vi "S7-PPI协议.vi"() -> ()   [LabVIEW 2014]
uses:
  <vilib>/Platform/browser.llb/Open URL in Default Browser (string).vi
  <vilib>/Instr/_visa.llb/VISA Configure Serial Port (Instr).vi
panel:
  out "RVW34":u16
  out "RVW32":u16
  out "RVW30":u16
  out "RVW28":u16
  out "RVW26":u16
  out "RVW24":u16
  out "RVW22":u16
  out "RVW20":u16
  out "RVW18":u16
  out "RVW16":u16
  out "RVW14":u16
  out "RVW12":u16
  out "RVW10":u16
  out "RVW8":u16
  out "RVW6":u16
  out "RVW4":u16
  out "RVW2":u16
  out "RVW0":u16
  in  "VW34":u16
  in  "VW32":u16
  in  "VW30":u16
  in  "VW28":u16
  in  "VW26":u16
  in  "VW24":u16
  in  "VW22":u16
  in  "VW20":u16
  in  "VW18":u16
  in  "VW16":u16
  in  "VW14":u16
  in  "VW12":u16
  in  "VW10":u16
  in  "VW8":u16
  in  "VW6":u16
  in  "VW4":u16
  in  "VW2":u16
  in  "VW0":u16
  out "值 3":u32
  out "Q3.0":bool
  out "Q3.1":bool
  out "Q3.2":bool
  out "Q3.3":bool
  out "Q3.4":bool
  out "Q3.5":bool
  out "Q3.6":bool
  out "Q3.7":bool
  out "M2.0":bool
  out "M2.1":bool
  out "M2.2":bool
  out "M2.4":bool
  out "M2.3":bool
  out "M2.5":bool
  out "M2.6":bool
  out "M2.7":bool
  out "M1.0":bool
  out "M1.1":bool
  out "M1.2":bool
  out "M1.3":bool
  out "M1.4":bool
  out "M1.5":bool
  out "M1.6":bool
  out "M1.7":bool
  out "M0.0":bool
  out "M0.1":bool
  out "M0.2":bool
  out "M0.3":bool
  out "M0.4":bool
  out "M0.5":bool
  out "M0.6":bool
  out "M0.7":bool
  in  "Q3.0":bool
  in  "Q3.1":bool
  in  "Q3.2":bool
  in  "Q3.3":bool
  in  "Q3.4":bool
  in  "Q3.5":bool
  in  "Q3.6":bool
  in  "Q3.7":bool
  in  "M2.0":bool
  in  "M2.1":bool
  in  "M2.2":bool
  in  "M2.3":bool
  in  "M2.4":bool
  in  "M2.5":bool
  in  "M2.6":bool
  in  "M2.7":bool
  in  "M1.0":bool
  in  "M1.1":bool
  in  "M1.2":bool
  in  "M1.3":bool
  in  "M1.4":bool
  in  "M1.5":bool
  in  "M1.6":bool
  in  "M1.7":bool
  in  "M0.0":bool
  in  "M0.1":bool
  in  "M0.2":bool
  in  "M0.3":bool
  in  "M0.4":bool
  in  "M0.5":bool
  in  "M0.6":bool
  in  "M0.7":bool
  out "值 2":u32
  in  "Q3.0":bool
  in  "Q3.1":bool
  in  "Q3.2":bool
  in  "Q3.3":bool
  in  "Q3.4":bool
  in  "Q3.5":bool
  in  "Q3.6":bool
  in  "Q3.7":bool
  in  "Q2.0":bool
  in  "Q2.1":bool
  in  "Q2.2":bool
  in  "Q2.3":bool
  in  "Q2.4":bool
  in  "Q2.5":bool
  in  "Q2.6":bool
  in  "Q2.7":bool
  in  "Q1.7":bool
  in  "Q1.6":bool
  in  "Q1.5":bool
  in  "Q1.4":bool
  in  "Q1.3":bool
  in  "Q1.2":bool
  in  "Q1.1":bool
  in  "Q1.0":bool
  in  "Q0.7":bool
  in  "Q0.6":bool
  in  "Q0.5":bool
  in  "Q0.4":bool
  in  "Q0.3":bool
  in  "Q0.2":bool
  in  "Q0.1":bool
  in  "Q0.0":bool
  out "Q3.0":bool
  out "Q3.1":bool
  out "Q3.2":bool
  out "Q3.3":bool
  out "Q3.4":bool
  out "Q3.5":bool
  out "Q3.6":bool
  out "Q3.7":bool
  out "Q2.0":bool
  out "Q2.1":bool
  out "Q2.2":bool
  out "Q2.4":bool
  out "Q2.3":bool
  out "Q2.5":bool
  out "Q2.6":bool
  out "Q2.7":bool
  out "Q1.0":bool
  out "Q1.1":bool
  out "Q1.2":bool
  out "Q1.3":bool
  out "Q1.4":bool
  out "Q1.5":bool
  out "Q1.6":bool
  out "Q1.7":bool
  out "Q0.0":bool
  out "Q0.1":bool
  out "Q0.2":bool
  out "Q0.3":bool
  out "Q0.4":bool
  out "Q0.5":bool
  out "Q0.6":bool
  out "Q0.7":bool
  out "I3.0":bool
  out "I3.1":bool
  out "I3.2":bool
  out "I3.3":bool
  out "I3.4":bool
  out "I3.5":bool
  out "I3.6":bool
  out "I3.7":bool
  out "I2.0":bool
  out "I2.1":bool
  out "I2.2":bool
  out "I2.4":bool
  out "I2.3":bool
  out "I2.5":bool
  out "I2.6":bool
  out "I2.7":bool
  out "I1.0":bool
  out "I1.1":bool
  out "I1.2":bool
  out "I1.3":bool
  out "I1.4":bool
  out "I1.5":bool
  out "I1.6":bool
  out "I1.7":bool
  out "I0.0":bool
  out "I0.1":bool
  out "I0.2":bool
  out "I0.3":bool
  out "I0.4":bool
  out "I0.5":bool
  out "I0.6":bool
  out "I0.7":bool
  in  "枚举":T1
  in  "读写时间":u32
  in  "baud":u32=9600 caption="波特率"
  in  "COM":refnum<visa-resource-name> caption="端口"
  in  "停止":bool
  in  "STOP":bool
  in  "RUN":bool
  # "I0.0-I0.7"
  # "I1.0-I1.7"
  # "I2.0-I2.7"
  # "I3.0-I3.7"
  # "https://item.taobao.com/item.htm?id=520867234520"
  # "Q0.0-Q0.7"
  # "Q1.0-Q1.7"
  # "Q2.0-Q2.7"
  # "Q3.0-Q3.7"
  # "本程序密码：635410@ ，已经由楼上的工具破解"
  # "M0.0-M0.7"
  # "M1.0-M1.7"
  # "M2.0-M2.7"
  # "M3.0-M3.7"
  # "运行前请选择正确的通讯端口，和\n波特率。注意读写扫描时间的填写\n此程序PLC默认地址为2，其他不能\n通讯连接。"
  # "注意：1:波特率19.2请将读写时间设置大于80，波特率9600请将读写时间设置大于200，禁止187.5运行,建议19.2kbt/s"
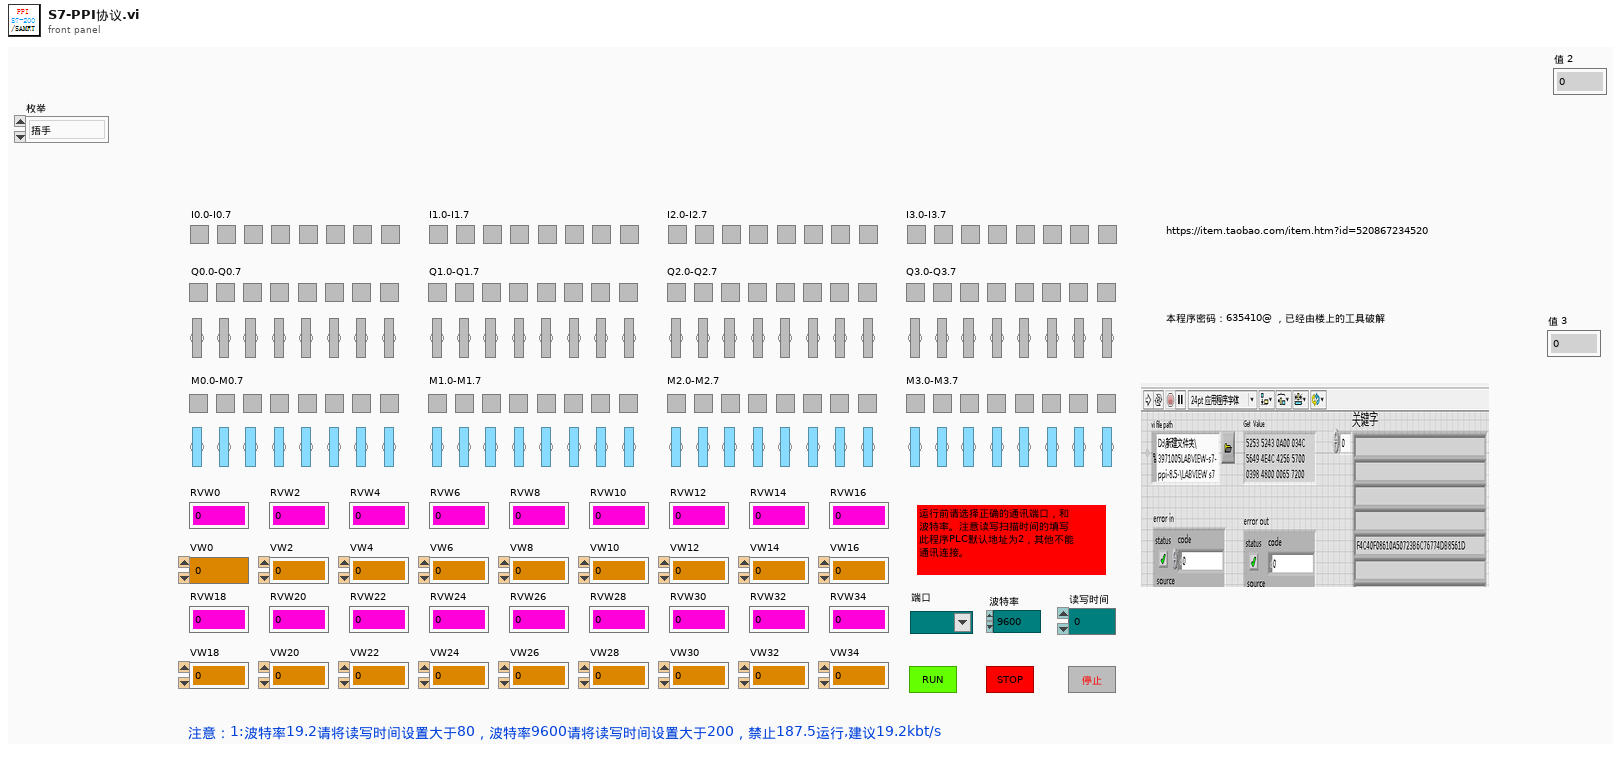
[diagram p1: front panel]
types:
  T1 = typedef "读取值枚举索引.ctl" = enum16{"捂手", "RUN", "STOP", "枚举RI", "枚举RQ", "枚举RM", "枚举RVW", "WID0", "WQD0", "WMD0", "WV"}
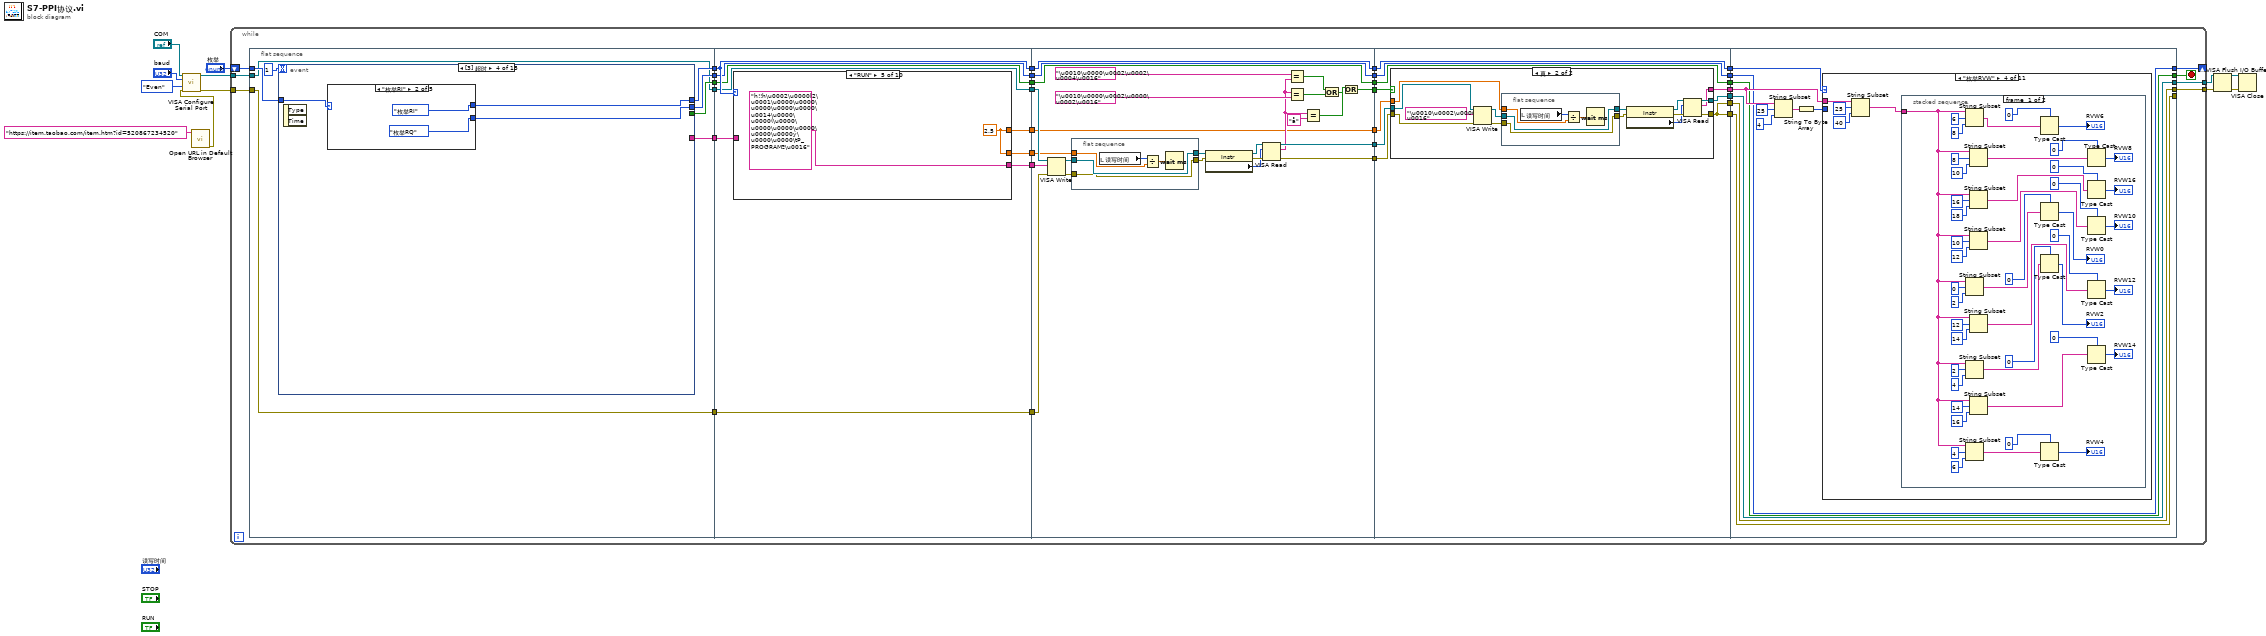
[diagram p0: block diagram]
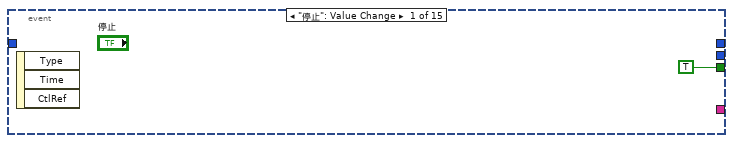
[diagram p2: hidden frame]
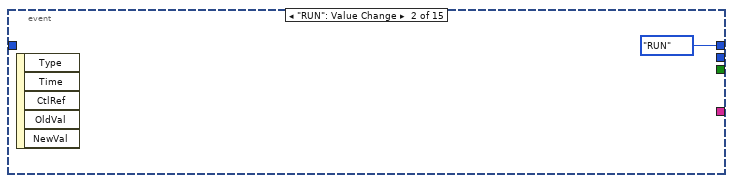
[diagram p3: hidden frame]
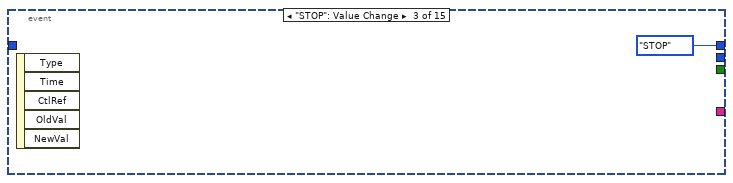
[diagram p4: hidden frame]
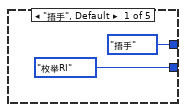
[diagram p5: hidden frame]
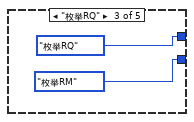
[diagram p6: hidden frame]
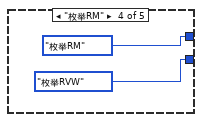
[diagram p7: hidden frame]
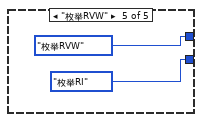
[diagram p8: hidden frame]
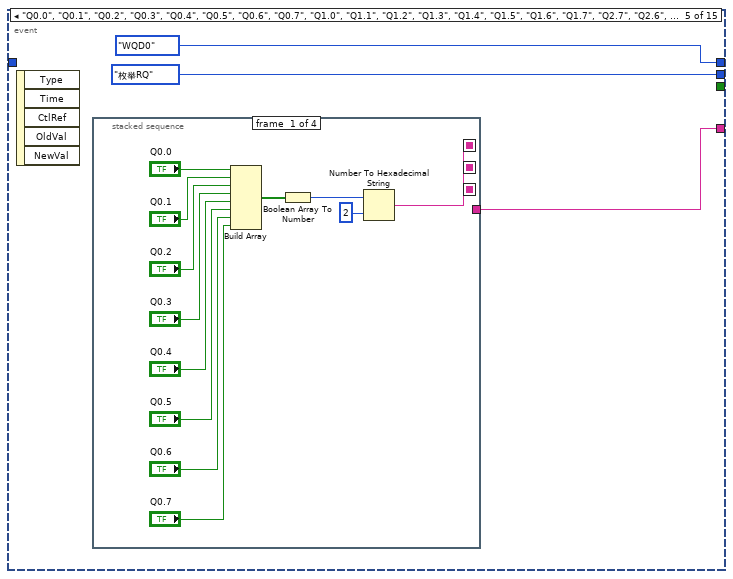
[diagram p9: hidden frame]
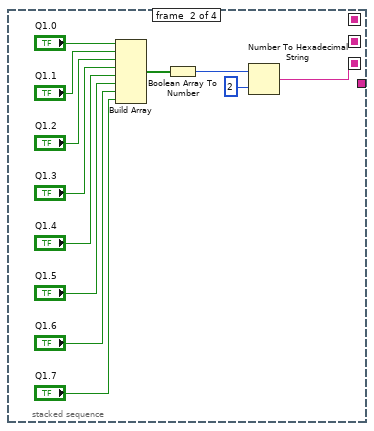
[diagram p10: hidden frame]
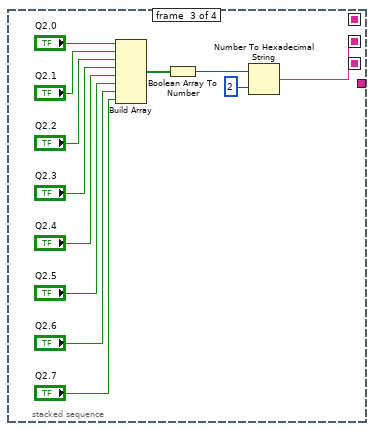
[diagram p11: hidden frame]
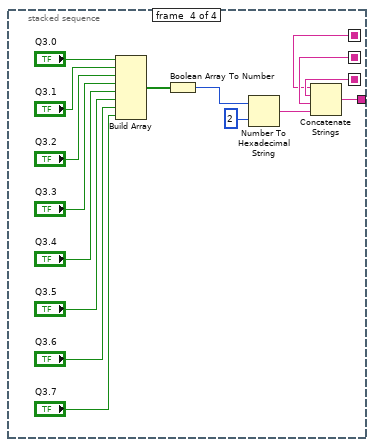
[diagram p12: hidden frame]
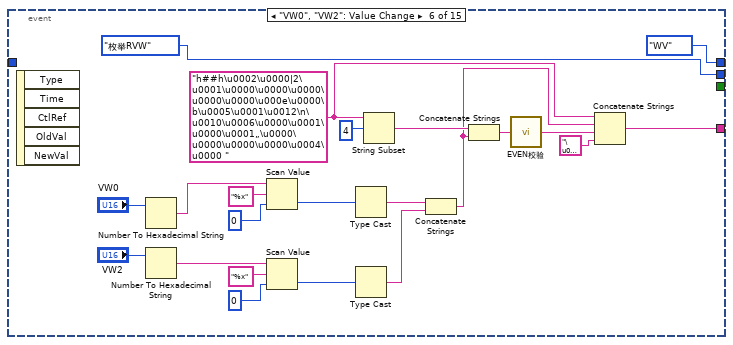
[diagram p13: hidden frame]
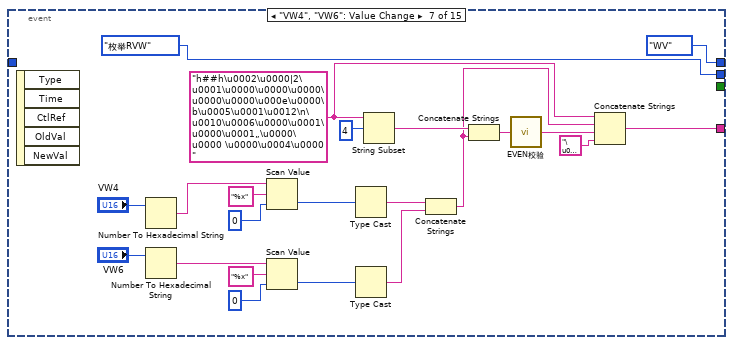
[diagram p14: hidden frame]
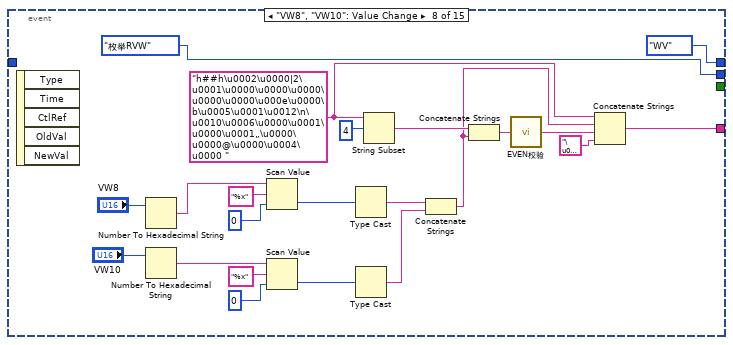
[diagram p15: hidden frame]
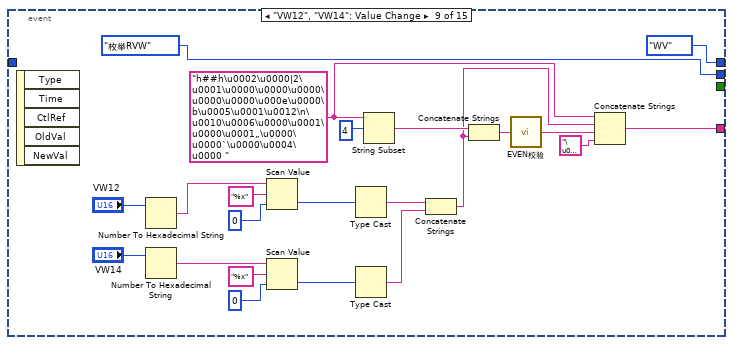
[diagram p16: hidden frame]
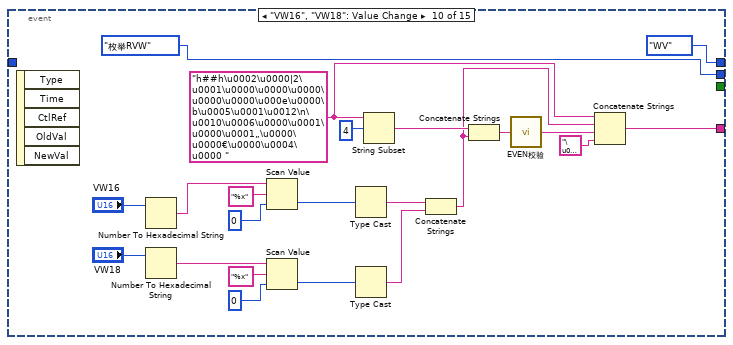
[diagram p17: hidden frame]
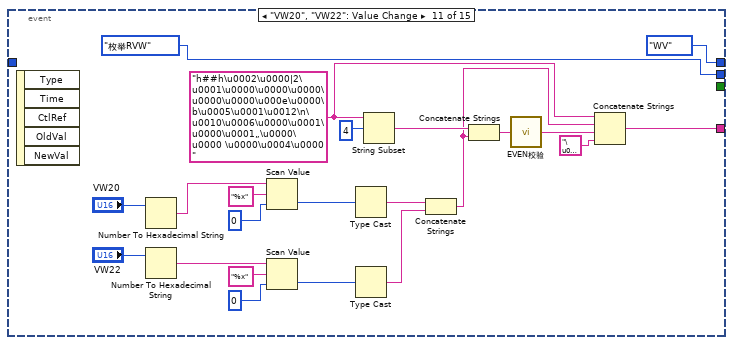
[diagram p18: hidden frame]
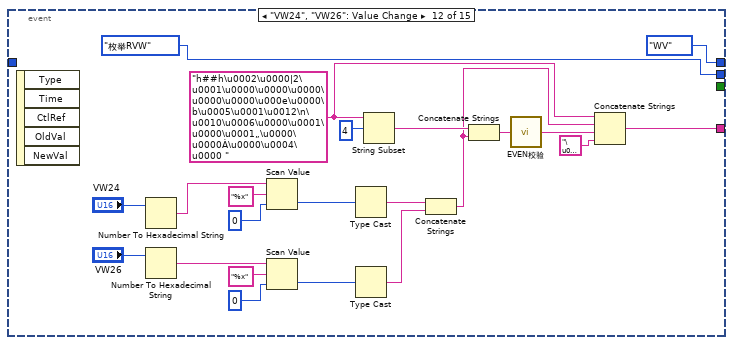
[diagram p19: hidden frame]
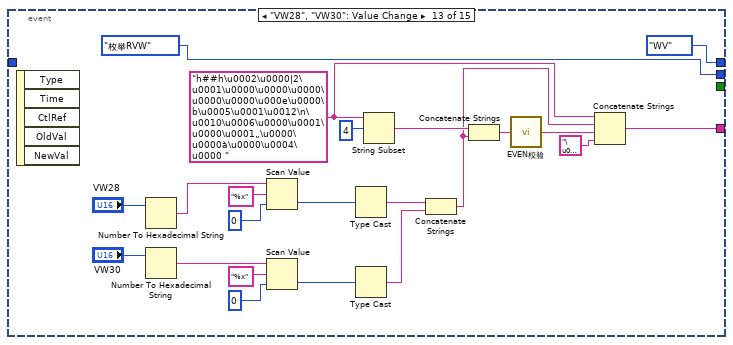
[diagram p20: hidden frame]
diagram:
  n1 = call-poly <vilib>:"Open URL in Default Browser.vi"("URL"="https://item.taobao.com/item.htm?id=520867234520") -> ("error out"=w1:errorcluster)  [unwired: 5 in, 1 out]
  n2 = call-poly "VISA Configure Serial Port"("VISA resource name"="COM", "baud rate (9600)"="baud", "parity (0:none)"=enum16{"None", "Odd", "Even", "Mark", "Space"}."Even", "error in (no error)"=w1) -> ("VISA resource name out"=w10:refnum<visa-resource-name>, "error out"=w9:errorcluster)  [unwired: 10 in]
  n3 = while {
    tunnel: w10 -> [w46]
    tunnel: w9 -> [w47]
    shift-right: [w44] -> _
    shift-left: "枚举" -> [w45]
    tunnel: [w42] -> w7
    tunnel: [w41] -> w6
    stop <- w43 stop-if-true
    n4 = flat-sequence {
      tunnel: w47 -> [w49]
      tunnel: w46 -> [w48]
      tunnel: w45 -> [w55]
      tunnel: [w49] -> w40
      tunnel: [w48] -> w39
      tunnel: [w54] -> w38
      tunnel: [w53] -> w37
      tunnel: [w52] -> w36
      tunnel: [w50] -> w35
      tunnel: w40 -> [w383]
      tunnel: w39 -> [w382]
      tunnel: w38 -> [w381]
      tunnel: w37 -> [w387]
      tunnel: w36 -> [w380]
      tunnel: w35 -> [w386]
      tunnel: [w383] -> w34
      tunnel: [w382] -> w33
      tunnel: [w381] -> w32
      tunnel: [w380] -> w31
      tunnel: [w388] -> w30
      tunnel: [w387] -> w29
      tunnel: [w385] -> w28
      tunnel: [w384] -> w27
      tunnel: w34 -> [w448]
      tunnel: w33 -> [w446]
      tunnel: w32 -> [w435]
      tunnel: w31 -> [w434]
      tunnel: w30 -> [w437]
      tunnel: w29 -> [w433]
      tunnel: w28 -> [w436]
      tunnel: w27 -> [w432]
      tunnel: [w435] -> w26
      tunnel: [w457] -> w25
      tunnel: [w456] -> w24
      tunnel: [w443] -> w23
      tunnel: [w434] -> w22
      tunnel: [w433] -> w21
      tunnel: [w432] -> w20
      tunnel: w26 -> [w464]
      tunnel: w25 -> [w471]
      tunnel: w24 -> [w470]
      tunnel: w23 -> [w472]
      tunnel: w22 -> [w465]
      tunnel: w21 -> [w463]
      tunnel: w20 -> [w466]
      tunnel: [w469] -> w19
      tunnel: [w468] -> w18
      tunnel: [w465] -> w17
      tunnel: [w464] -> w16
      tunnel: [w468] -> w15
      tunnel: [w467] -> w14
      tunnel: [w463] -> w13
      tunnel: [w498] -> w42
      tunnel: [w497] -> _
      tunnel: [w496] -> w44
      tunnel: [w495] -> w43
      tunnel: [w494] -> w41
      tunnel: w19 -> [w498]
      tunnel: w18 -> [w497]
      tunnel: w17 -> [w496]
      tunnel: w16 -> [w495]
      tunnel: w15 -> [w494]
      tunnel: w14 -> [w499]
      tunnel: w13 -> [w500]
      frame #0 {
        n5 = event shown="[3] 超时" {
          selector: _ -> [_ _ _ _ _ _ _ _ _ _ _ _ _ _ _]
          dyn-events: _ -> [_ _ _ _ _ _ _ _ _ _ _ _ _ _ _]
          timeout: 1 -> [_ _ _ _ _ _ _ _ _ _ _ _ _ _ _]
          tunnel: w55 -> [_ _ _ w61 _ _ _ _ _ _ _ _ _ _ _]
          tunnel: [_ 读取值枚举索引."RUN" ("枚举 2") 读取值枚举索引."STOP" ("枚举 2") w60 读取值枚举索引."WQD0" ("枚举 2") 读取值枚举索引."WV" ("枚举 2") 读取值枚举索引."WV" ("枚举 2") 读取值枚举索引."WV" ("枚举 2") 读取值枚举索引."WV" ("枚举 2") 读取值枚举索引."WV" ("枚举 2") 读取值枚举索引."WV" ("枚举 2") 读取值枚举索引."WV" ("枚举 2") 读取值枚举索引."WV" ("枚举 2") 读取值枚举索引."WV" ("枚举 2") 读取值枚举索引."WMD0" ("枚举 2")] -> w53
          tunnel: [TRUE _ _ _ _ _ _ _ _ _ _ _ _ _ _] -> w54
          tunnel: [_ _ _ w59 读取值枚举索引."枚举RQ" ("枚举 2") 读取值枚举索引."枚举RVW" ("枚举 2") 读取值枚举索引."枚举RVW" ("枚举 2") 读取值枚举索引."枚举RVW" ("枚举 2") 读取值枚举索引."枚举RVW" ("枚举 2") 读取值枚举索引."枚举RVW" ("枚举 2") 读取值枚举索引."枚举RVW" ("枚举 2") 读取值枚举索引."枚举RVW" ("枚举 2") 读取值枚举索引."枚举RVW" ("枚举 2") 读取值枚举索引."枚举RVW" ("枚举 2") 读取值枚举索引."枚举RM" ("枚举 2")] -> w52
          tunnel: [_ _ _ _ w72 w133 w155 w177 w199 w222 w243 w265 w285 w308 w327] -> w50
          event "停止": Value Change {
            n6 = event-data() -> ()  [unwired: 1 in, 3 out]
          }
          event "RUN": Value Change {
            n7 = event-data() -> ()  [unwired: 1 in, 5 out]
          }
          event "STOP": Value Change {
            n8 = event-data() -> ()  [unwired: 1 in, 5 out]
          }
          event Timeout {
            n9 = event-data() -> ()  [unwired: 1 in, 2 out]
            n10 = case shown="\"枚举RI\"" w61 {
              tunnel: [读取值枚举索引."捂手" ("枚举 2") 读取值枚举索引."枚举RI" ("枚举 2") 读取值枚举索引."枚举RQ" ("枚举 2") 读取值枚举索引."枚举RM" ("枚举 2") 读取值枚举索引."枚举RVW" ("枚举 2")] -> w60
              tunnel: [读取值枚举索引."枚举RI" ("枚举 2") 读取值枚举索引."枚举RQ" ("枚举 2") 读取值枚举索引."枚举RM" ("枚举 2") 读取值枚举索引."枚举RVW" ("枚举 2") 读取值枚举索引."枚举RI" ("枚举 2")] -> w59
              frame "捂手", Default {
              }
              frame "枚举RI" {
              }
              frame "枚举RQ" {
              }
              frame "枚举RM" {
              }
              frame "枚举RVW" {
              }
            }
          }
          event "Q0.0", "Q0.1", "Q0.2", "Q0.3", "Q0.4", "Q0.5", "Q0.6", "Q0.7", "Q1.0", "Q1.1", "Q1.2", "Q1.3", "Q1.4", "Q1.5", "Q1.6", "Q1.7", "Q2.7", "Q2.6", "Q2.5", "Q2.4", "Q2.3", "Q2.2", "Q2.1", "Q2.0", "Q3.7", "Q3.5", "Q3.4", "Q3.3", "Q3.2", "Q3.1", "Q3.0": Value Change {
            n11 = event-data() -> ()  [unwired: 1 in, 5 out]
            n12 = stacked-sequence {
              seq-local: [w75 _ _ _] -> [_ _ _ w112]
              seq-local: [_ w87 _ _] -> [_ _ _ w115]
              seq-local: [_ _ w99 _] -> [_ _ _ w114]
              tunnel: [_ _ _ w111] -> w72
              frame #0 {
                n13 = Build Array("Q0.0", "Q0.1", "Q0.2", "Q0.3", "Q0.4", "Q0.5", "Q0.6", "Q0.7") -> (w86:bool[])
                n14 = Boolean Array To Number(Boolean array=w86) -> (number=w84:u32)
                n15 = Number To Hexadecimal String(1:i16 2 ("宽度(-)"), 2:w84) -> (0:w75:string)
              }
              frame #1 {
                n16 = Build Array("Q1.0", "Q1.1", "Q1.2", "Q1.3", "Q1.4", "Q1.5", "Q1.6", "Q1.7") -> (w98:bool[])
                n17 = Boolean Array To Number(Boolean array=w98) -> (number=w96:u32)
                n18 = Number To Hexadecimal String(1:i16 2 ("宽度(-)"), 2:w96) -> (0:w87:string)
              }
              frame #2 {
                n19 = Build Array("Q2.0", "Q2.1", "Q2.2", "Q2.3", "Q2.4", "Q2.5", "Q2.6", "Q2.7") -> (w110:bool[])
                n20 = Boolean Array To Number(Boolean array=w110) -> (number=w108:u32)
                n21 = Number To Hexadecimal String(1:i16 2 ("宽度(-)"), 2:w108) -> (0:w99:string)
              }
              frame #3 {
                n22 = Build Array("Q3.0", "Q3.1", "Q3.2", "Q3.3", "Q3.4", "Q3.5", "Q3.6", "Q3.7") -> (w124:bool[])
                n23 = Boolean Array To Number(Boolean array=w124) -> (number=w126:u32)
                n24 = Number To Hexadecimal String(1:i16 2 ("宽度(-)"), 2:w126) -> (0:w113:string)
                n25 = Concatenate Strings(w112, w115, w114, w113) -> (w111:string)
              }
            }
          }
          event "VW0", "VW2": Value Change {
            w128 = "h##h\u0002\u0000|2\u0001\u0000\u0000\u0000\u0000\u0000\u000e\u0000\b\u0005\u0001\u0012\n\u0010\u0006\u0000\u0001\u0000\u0001„\u0000\u0000\u0000\u0000\u0004\u0000 "
            n26 = event-data() -> ()  [unwired: 1 in, 5 out]
            n27 = Number To Hexadecimal String(2:"VW0") -> (0:w143:string)  [unwired: 1 in]
            n28 = Number To Hexadecimal String(2:"VW2") -> (0:w148:string)  [unwired: 1 in]
            n29 = Scan Value(string=w143, format string="%x" ("格式字符串"), default (0 dbl)=u16 0 ("默认(0 dbl)")) -> (value=w144:u16)  [unwired: 1 out]
            n30 = Scan Value(string=w148, format string="%x" ("格式字符串"), default (0 dbl)=u16 0 ("默认(0 dbl)")) -> (value=w145:u16)  [unwired: 1 out]
            n31 = Type Cast(x=w144) -> (*(type *) &x=w130:string)  [unwired: 1 in]
            n32 = Type Cast(x=w145) -> (*(type *) &x=w129:string)  [unwired: 1 in]
            n33 = String Subset(string=w128, offset (0)=4 ("偏移量(0)")) -> (substring=w137:string)  [unwired: 1 in]
            n34 = Concatenate Strings(w130, w129) -> (w127:string)
            n35 = Concatenate Strings(w137, w127) -> (w134:string)
            n36 = call "EVEN校验.vi"("校验字符串"=w134) -> ("校验码"=w136:string)
            n37 = Concatenate Strings(w128, w127, w136, "\u0016" ("字符串")) -> (w133:string)
          }
          event "VW4", "VW6": Value Change {
            w152 = "h##h\u0002\u0000|2\u0001\u0000\u0000\u0000\u0000\u0000\u000e\u0000\b\u0005\u0001\u0012\n\u0010\u0006\u0000\u0001\u0000\u0001„\u0000\u0000 \u0000\u0004\u0000 "
            n38 = event-data() -> ()  [unwired: 1 in, 5 out]
            n39 = Number To Hexadecimal String(2:"VW4") -> (0:w170:string)  [unwired: 1 in]
            n40 = Number To Hexadecimal String(2:"VW6") -> (0:w165:string)  [unwired: 1 in]
            n41 = Scan Value(string=w170, format string="%x" ("格式字符串"), default (0 dbl)=u16 0 ("默认(0 dbl)")) -> (value=w167:u16)  [unwired: 1 out]
            n42 = Scan Value(string=w165, format string="%x" ("格式字符串"), default (0 dbl)=u16 0 ("默认(0 dbl)")) -> (value=w166:u16)  [unwired: 1 out]
            n43 = Type Cast(x=w167) -> (*(type *) &x=w149:string)  [unwired: 1 in]
            n44 = Type Cast(x=w166) -> (*(type *) &x=w150:string)  [unwired: 1 in]
            n45 = String Subset(string=w152, offset (0)=4 ("偏移量(0)")) -> (substring=w161:string)  [unwired: 1 in]
            n46 = Concatenate Strings(w149, w150) -> (w151:string)
            n47 = Concatenate Strings(w161, w151) -> (w158:string)
            n48 = call "EVEN校验.vi"("校验字符串"=w158) -> ("校验码"=w160:string)
            n49 = Concatenate Strings(w152, w151, w160, "\u0016" ("字符串")) -> (w155:string)
          }
          event "VW8", "VW10": Value Change {
            w174 = "h##h\u0002\u0000|2\u0001\u0000\u0000\u0000\u0000\u0000\u000e\u0000\b\u0005\u0001\u0012\n\u0010\u0006\u0000\u0001\u0000\u0001„\u0000\u0000@\u0000\u0004\u0000 "
            n50 = event-data() -> ()  [unwired: 1 in, 5 out]
            n51 = Number To Hexadecimal String(2:"VW8") -> (0:w192:string)  [unwired: 1 in]
            n52 = Number To Hexadecimal String(2:"VW10") -> (0:w187:string)  [unwired: 1 in]
            n53 = Scan Value(string=w192, format string="%x" ("格式字符串"), default (0 dbl)=u16 0 ("默认(0 dbl)")) -> (value=w189:u16)  [unwired: 1 out]
            n54 = Scan Value(string=w187, format string="%x" ("格式字符串"), default (0 dbl)=u16 0 ("默认(0 dbl)")) -> (value=w188:u16)  [unwired: 1 out]
            n55 = Type Cast(x=w189) -> (*(type *) &x=w171:string)  [unwired: 1 in]
            n56 = Type Cast(x=w188) -> (*(type *) &x=w172:string)  [unwired: 1 in]
            n57 = String Subset(string=w174, offset (0)=4 ("偏移量(0)")) -> (substring=w183:string)  [unwired: 1 in]
            n58 = Concatenate Strings(w171, w172) -> (w173:string)
            n59 = Concatenate Strings(w183, w173) -> (w180:string)
            n60 = call "EVEN校验.vi"("校验字符串"=w180) -> ("校验码"=w182:string)
            n61 = Concatenate Strings(w174, w173, w182, "\u0016" ("字符串")) -> (w177:string)
          }
          event "VW12", "VW14": Value Change {
            w196 = "h##h\u0002\u0000|2\u0001\u0000\u0000\u0000\u0000\u0000\u000e\u0000\b\u0005\u0001\u0012\n\u0010\u0006\u0000\u0001\u0000\u0001„\u0000\u0000`\u0000\u0004\u0000 "
            n62 = event-data() -> ()  [unwired: 1 in, 5 out]
            n63 = Number To Hexadecimal String(2:"VW12") -> (0:w214:string)  [unwired: 1 in]
            n64 = Number To Hexadecimal String(2:"VW14") -> (0:w209:string)  [unwired: 1 in]
            n65 = Scan Value(string=w214, format string="%x" ("格式字符串"), default (0 dbl)=u16 0 ("默认(0 dbl)")) -> (value=w211:u16)  [unwired: 1 out]
            n66 = Scan Value(string=w209, format string="%x" ("格式字符串"), default (0 dbl)=u16 0 ("默认(0 dbl)")) -> (value=w210:u16)  [unwired: 1 out]
            n67 = Type Cast(x=w211) -> (*(type *) &x=w194:string)  [unwired: 1 in]
            n68 = Type Cast(x=w210) -> (*(type *) &x=w193:string)  [unwired: 1 in]
            n69 = String Subset(string=w196, offset (0)=4 ("偏移量(0)")) -> (substring=w205:string)  [unwired: 1 in]
            n70 = Concatenate Strings(w194, w193) -> (w195:string)
            n71 = Concatenate Strings(w205, w195) -> (w202:string)
            n72 = call "EVEN校验.vi"("校验字符串"=w202) -> ("校验码"=w204:string)
            n73 = Concatenate Strings(w196, w195, w204, "\u0016" ("字符串")) -> (w199:string)
          }
          event "VW16", "VW18": Value Change {
            w217 = "h##h\u0002\u0000|2\u0001\u0000\u0000\u0000\u0000\u0000\u000e\u0000\b\u0005\u0001\u0012\n\u0010\u0006\u0000\u0001\u0000\u0001„\u0000\u0000€\u0000\u0004\u0000 "
            n74 = event-data() -> ()  [unwired: 1 in, 5 out]
            n75 = Number To Hexadecimal String(2:"VW16") -> (0:w231:string)  [unwired: 1 in]
            n76 = Number To Hexadecimal String(2:"VW18") -> (0:w236:string)  [unwired: 1 in]
            n77 = Scan Value(string=w231, format string="%x" ("格式字符串"), default (0 dbl)=u16 0 ("默认(0 dbl)")) -> (value=w232:u16)  [unwired: 1 out]
            n78 = Scan Value(string=w236, format string="%x" ("格式字符串"), default (0 dbl)=u16 0 ("默认(0 dbl)")) -> (value=w233:u16)  [unwired: 1 out]
            n79 = Type Cast(x=w232) -> (*(type *) &x=w219:string)  [unwired: 1 in]
            n80 = Type Cast(x=w233) -> (*(type *) &x=w218:string)  [unwired: 1 in]
            n81 = String Subset(string=w217, offset (0)=4 ("偏移量(0)")) -> (substring=w227:string)  [unwired: 1 in]
            n82 = Concatenate Strings(w219, w218) -> (w215:string)
            n83 = Concatenate Strings(w227, w215) -> (w216:string)
            n84 = call "EVEN校验.vi"("校验字符串"=w216) -> ("校验码"=w226:string)
            n85 = Concatenate Strings(w217, w215, w226, "\u0016" ("字符串")) -> (w222:string)
          }
          event "VW20", "VW22": Value Change {
            w240 = "h##h\u0002\u0000|2\u0001\u0000\u0000\u0000\u0000\u0000\u000e\u0000\b\u0005\u0001\u0012\n\u0010\u0006\u0000\u0001\u0000\u0001„\u0000\u0000 \u0000\u0004\u0000 "
            n86 = event-data() -> ()  [unwired: 1 in, 5 out]
            n87 = Number To Hexadecimal String(2:"VW20") -> (0:w258:string)  [unwired: 1 in]
            n88 = Number To Hexadecimal String(2:"VW22") -> (0:w253:string)  [unwired: 1 in]
            n89 = Scan Value(string=w258, format string="%x" ("格式字符串"), default (0 dbl)=u16 0 ("默认(0 dbl)")) -> (value=w255:u16)  [unwired: 1 out]
            n90 = Scan Value(string=w253, format string="%x" ("格式字符串"), default (0 dbl)=u16 0 ("默认(0 dbl)")) -> (value=w254:u16)  [unwired: 1 out]
            n91 = Type Cast(x=w255) -> (*(type *) &x=w237:string)  [unwired: 1 in]
            n92 = Type Cast(x=w254) -> (*(type *) &x=w238:string)  [unwired: 1 in]
            n93 = String Subset(string=w240, offset (0)=4 ("偏移量(0)")) -> (substring=w249:string)  [unwired: 1 in]
            n94 = Concatenate Strings(w237, w238) -> (w239:string)
            n95 = Concatenate Strings(w249, w239) -> (w246:string)
            n96 = call "EVEN校验.vi"("校验字符串"=w246) -> ("校验码"=w248:string)
            n97 = Concatenate Strings(w240, w239, w248, "\u0016" ("字符串")) -> (w243:string)
          }
          event "VW24", "VW26": Value Change {
            w260 = "h##h\u0002\u0000|2\u0001\u0000\u0000\u0000\u0000\u0000\u000e\u0000\b\u0005\u0001\u0012\n\u0010\u0006\u0000\u0001\u0000\u0001„\u0000\u0000À\u0000\u0004\u0000 "
            n98 = event-data() -> ()  [unwired: 1 in, 5 out]
            n99 = Number To Hexadecimal String(2:"VW24") -> (0:w275:string)  [unwired: 1 in]
            n100 = Number To Hexadecimal String(2:"VW26") -> (0:w280:string)  [unwired: 1 in]
            n101 = Scan Value(string=w275, format string="%x" ("格式字符串"), default (0 dbl)=u16 0 ("默认(0 dbl)")) -> (value=w276:u16)  [unwired: 1 out]
            n102 = Scan Value(string=w280, format string="%x" ("格式字符串"), default (0 dbl)=u16 0 ("默认(0 dbl)")) -> (value=w277:u16)  [unwired: 1 out]
            n103 = Type Cast(x=w276) -> (*(type *) &x=w262:string)  [unwired: 1 in]
            n104 = Type Cast(x=w277) -> (*(type *) &x=w261:string)  [unwired: 1 in]
            n105 = String Subset(string=w260, offset (0)=4 ("偏移量(0)")) -> (substring=w271:string)  [unwired: 1 in]
            n106 = Concatenate Strings(w262, w261) -> (w259:string)
            n107 = Concatenate Strings(w271, w259) -> (w268:string)
            n108 = call "EVEN校验.vi"("校验字符串"=w268) -> ("校验码"=w270:string)
            n109 = Concatenate Strings(w260, w259, w270, "\u0016" ("字符串")) -> (w265:string)
          }
          event "VW28", "VW30": Value Change {
            w282 = "h##h\u0002\u0000|2\u0001\u0000\u0000\u0000\u0000\u0000\u000e\u0000\b\u0005\u0001\u0012\n\u0010\u0006\u0000\u0001\u0000\u0001„\u0000\u0000à\u0000\u0004\u0000 "
            n110 = event-data() -> ()  [unwired: 1 in, 5 out]
            n111 = Number To Hexadecimal String(2:"VW28") -> (0:w295:string)  [unwired: 1 in]
            n112 = Number To Hexadecimal String(2:"VW30") -> (0:w290:string)  [unwired: 1 in]
            n113 = Scan Value(string=w295, format string="%x" ("格式字符串"), default (0 dbl)=u16 0 ("默认(0 dbl)")) -> (value=w294:u16)  [unwired: 1 out]
            n114 = Scan Value(string=w290, format string="%x" ("格式字符串"), default (0 dbl)=u16 0 ("默认(0 dbl)")) -> (value=w293:u16)  [unwired: 1 out]
            n115 = Type Cast(x=w294) -> (*(type *) &x=w284:string)  [unwired: 1 in]
            n116 = Type Cast(x=w293) -> (*(type *) &x=w283:string)  [unwired: 1 in]
            n117 = String Subset(string=w282, offset (0)=4 ("偏移量(0)")) -> (substring=w299:string)  [unwired: 1 in]
            n118 = Concatenate Strings(w284, w283) -> (w281:string)
            n119 = Concatenate Strings(w299, w281) -> (w302:string)
            n120 = call "EVEN校验.vi"("校验字符串"=w302) -> ("校验码"=w300:string)
            n121 = Concatenate Strings(w282, w281, w300, "\u0016" ("字符串")) -> (w285:string)
          }
          event "VW32", "VW34": Value Change {
            w304 = "h##h\u0002\u0000|2\u0001\u0000\u0000\u0000\u0000\u0000\u000e\u0000\b\u0005\u0001\u0012\n\u0010\u0006\u0000\u0001\u0000\u0001„\u0000\u0001\u0000\u0000\u0004\u0000 "
            n122 = event-data() -> ()  [unwired: 1 in, 5 out]
            n123 = Number To Hexadecimal String(2:"VW32") -> (0:w319:string)  [unwired: 1 in]
            n124 = Number To Hexadecimal String(2:"VW34") -> (0:w324:string)  [unwired: 1 in]
            n125 = Scan Value(string=w319, format string="%x" ("格式字符串"), default (0 dbl)=u16 0 ("默认(0 dbl)")) -> (value=w320:u16)  [unwired: 1 out]
            n126 = Scan Value(string=w324, format string="%x" ("格式字符串"), default (0 dbl)=u16 0 ("默认(0 dbl)")) -> (value=w321:u16)  [unwired: 1 out]
            n127 = Type Cast(x=w320) -> (*(type *) &x=w307:string)  [unwired: 1 in]
            n128 = Type Cast(x=w321) -> (*(type *) &x=w306:string)  [unwired: 1 in]
            n129 = String Subset(string=w304, offset (0)=4 ("偏移量(0)")) -> (substring=w316:string)  [unwired: 1 in]
            n130 = Concatenate Strings(w307, w306) -> (w303:string)
            n131 = Concatenate Strings(w316, w303) -> (w313:string)
            n132 = call "EVEN校验.vi"("校验字符串"=w313) -> ("校验码"=w315:string)
            n133 = Concatenate Strings(w304, w303, w315, "\u0016" ("字符串")) -> (w308:string)
          }
          event "M1.7", "M0.6", "M0.5", "M0.4", "M0.3", "M0.2", "M0.1", "M0.0", "M1.6", "M1.5", "M1.4", "M1.3", "M1.2", "M1.1", "M0.7", "M1.0", "M2.7", "M2.6", "M2.5", "M2.4", "M2.3", "M2.2", "M2.1", "M2.0", "Q3.7", "Q3.6", "Q3.5", "Q3.4", "Q3.3", "Q3.2", "Q3.1", "Q3.0": Value Change {
            n134 = event-data() -> ()  [unwired: 1 in, 5 out]
            n135 = stacked-sequence {
              seq-local: [w328 _ _ _] -> [_ _ _ w365]
              seq-local: [_ w340 _ _] -> [_ _ _ w368]
              seq-local: [_ _ w352 _] -> [_ _ _ w367]
              tunnel: [_ _ _ w364] -> w327
              frame #0 {
                n136 = Build Array("M0.0", "M0.1", "M0.2", "M0.3", "M0.4", "M0.5", "M0.6", "M0.7") -> (w339:bool[])
                n137 = Boolean Array To Number(Boolean array=w339) -> (number=w337:u32)
                n138 = Number To Hexadecimal String(1:i16 2 ("宽度(-)"), 2:w337) -> (0:w328:string)
              }
              frame #1 {
                n139 = Build Array("M1.0", "M1.1", "M1.2", "M1.3", "M1.4", "M1.5", "M1.6", "M1.7") -> (w351:bool[])
                n140 = Boolean Array To Number(Boolean array=w351) -> (number=w349:u32)
                n141 = Number To Hexadecimal String(1:i16 2 ("宽度(-)"), 2:w349) -> (0:w340:string)
              }
              frame #2 {
                n142 = Build Array("M2.0", "M2.1", "M2.2", "M2.3", "M2.4", "M2.5", "M2.6", "M2.7") -> (w363:bool[])
                n143 = Boolean Array To Number(Boolean array=w363) -> (number=w361:u32)
                n144 = Number To Hexadecimal String(1:i16 2 ("宽度(-)"), 2:w361) -> (0:w352:string)
              }
              frame #3 {
                n145 = Build Array("Q3.0", "Q3.1", "Q3.2", "Q3.3", "Q3.4", "Q3.5", "Q3.6", "Q3.7") -> (w377:bool[])
                n146 = Boolean Array To Number(Boolean array=w377) -> (number=w379:u32)
                n147 = Number To Hexadecimal String(1:i16 2 ("宽度(-)"), 2:w379) -> (0:w366:string)
                n148 = Concatenate Strings(w365, w368, w367, w366) -> (w364:string)
              }
            }
          }
        }
      }
      frame #1 {
        n149 = case shown="\"RUN\"" w387 {
          tunnel: ["\u0010\u0002\u0000IK\u0016" ("写入缓冲区") "h\u001b\u001bh\u0002\u0000l2\u0001\u0000\u0000\u0000\u0000\u0000\u000e\u0000\u0000\u0004\u0001\u0012\n\u0010\u0006\u0000\u0001\u0000\u0000\u0000\u0000\u0000h\u0016" ("写入缓冲区") "h\u001b\u001bh\u0002\u0000l2\u0001\u0000\u0000\u0000\u0000\u0000\u000e\u0000\u0000\u0004\u0001\u0012\n\u0010\u0006\u0000\u0001\u0000\u0000‚\u0000\u0000\u0000i\u0016" ("写入缓冲区") "h\u001b\u001bh\u0002\u0000l2\u0001\u0000\u0000\u0000\u0000\u0000\u000e\u0000\u0000\u0004\u0001\u0012\n\u0010\u0006\u0000\u0001\u0000\u0000ƒ\u0000\u0000\u0000j\u0016" ("写入缓冲区") "h!!h\u0002\u0000l2\u0001\u0000\u0000\u0000\u0000\u0000\u0014\u0000\u0000(\u0000\u0000\u0000\u0000\u0000\u0000ý\u0000\u0000\tP_PROGRAMª\u0016" "h\u001d\u001dh\u0002\u0000l2\u0001\u0000\u0000\u0000\u0000\u0000\u0010\u0000\u0000)\u0000\u0000\u0000\u0000\u0000\tP_PROGRAMª\u0016" w407 w415 w428 "h\u001b\u001bh\u0002\u0000l2\u0001\u0000\u0000\u0000\u0000\u0000\u000e\u0000\u0000\u0004\u0001\u0012\n\u0010\u0006\u0000\n\u0000\u0001„\u0000\u0000\u0000u\u0016" ("写入缓冲区")] -> w388
          tunnel: w386 -> [_ _ _ _ _ _ w403 w416 w428 _]
          tunnel: [w389 w391 w393 w395 w397 w399 w401 w414 w427 2.0 ("y")] -> w385
          tunnel: [w389 w391 w393 w395 w397 w399 w401 w414 w427 1.0 ("y")] -> w384
          frame "捂手", Default {
            w389 = 2.5 ("y")
          }
          frame "枚举RI" {
            w391 = 2.5 ("y")
          }
          frame "枚举RQ" {
            w393 = 2.5 ("y")
          }
          frame "枚举RM" {
            w395 = 2.5 ("y")
          }
          frame "RUN" {
            w397 = 2.5 ("y")
          }
          frame "STOP" {
            w399 = 2.5 ("y")
          }
          frame "WQD0" {
            w401 = 2.5 ("y")
            w410 = "h##h\u0002\u0000|2\u0001\u0000\u0000\u0000\u0000\u0000\u000e\u0000\b\u0005\u0001\u0012\n\u0010\u0006\u0000\u0001\u0000\u0000‚\u0000\u0000\u0000\u0000\u0004\u0000 "
            n150 = Scan Value(string=w403, format string="%x" ("格式字符串"), default (0 dbl)=u32 0 ("默认(0 dbl)")) -> (value=w406:u32)  [unwired: 1 out]
            "值 2" <- w406
            n151 = Type Cast(x=w406) -> (*(type *) &x=w402:string)  [unwired: 1 in]
            n152 = String Subset(string=w410, offset (0)=4 ("偏移量(0)")) -> (substring=w412:string)  [unwired: 1 in]
            n153 = Concatenate Strings(w412, w402) -> (w411:string)
            n154 = call "EVEN校验.vi"("校验字符串"=w411) -> ("校验码"=w409:string)
            n155 = Concatenate Strings(w410, w402, w409, "\u0016" ("字符串")) -> (w407:string)
          }
          frame "WMD0" {
            w414 = 2.5 ("y")
            w423 = "h##h\u0002\u0000|2\u0001\u0000\u0000\u0000\u0000\u0000\u000e\u0000\b\u0005\u0001\u0012\n\u0010\u0006\u0000\u0001\u0000\u0000ƒ\u0000\u0000\u0000\u0000\u0004\u0000 "
            n156 = Scan Value(string=w416, format string="%x" ("格式字符串"), default (0 dbl)=u32 0 ("默认(0 dbl)")) -> (value=w420:u32)  [unwired: 1 out]
            "值 3" <- w420
            n157 = Type Cast(x=w420) -> (*(type *) &x=w417:string)  [unwired: 1 in]
            n158 = String Subset(string=w423, offset (0)=4 ("偏移量(0)")) -> (substring=w425:string)  [unwired: 1 in]
            n159 = Concatenate Strings(w425, w417) -> (w424:string)
            n160 = call "EVEN校验.vi"("校验字符串"=w424) -> ("校验码"=w422:string)
            n161 = Concatenate Strings(w423, w417, w422, "\u0016" ("字符串")) -> (w415:string)
          }
          frame "WV" {
            w427 = 2.5 ("y")
          }
          frame "枚举RVW" {
          }
        }
      }
      frame #2 {
        n162 = VISA Write(VISA resource name=w446, write buffer=w437, error in (no error)=w448) -> (VISA resource name out=w452:refnum<visa-resource-name>, error out=w449:errorcluster)  [unwired: 1 out]
        n163 = flat-sequence {
          tunnel: w452 -> [w460]
          tunnel: [w460] -> w451
          tunnel: [w459] -> w450
          tunnel: w449 -> [w459]
          tunnel: w436 -> [w458]
          frame #0 {
            n164 = local read "读写时间"() -> (w461:u32)
            n165 = Divide(x=w461, y=w458) -> (x/y=w462:dbl)
            n166 = Wait (ms)(milliseconds to wait=w462) -> ()  [unwired: 1 out]
          }
        }
        n167 = property class="Instr"(reference=w451, error in=w450) -> (reference out=w453:refnum<visa-resource-name>, error out=w455:errorcluster, "Serial Settings:Number of Bytes at Serial Port"=w454:u32)
        n168 = VISA Read(VISA resource name=w453, byte count=w454, error in (no error)=w455) -> (VISA resource name out=w457:refnum<visa-resource-name>, read buffer=w442:string, error out=w456:errorcluster)  [unwired: 1 out]
        n169 = Equal?(x="\u0010\u0000\u0002\u0002\u0004\u0016" ("y"), y=w442) -> (x = y?=w440:bool)
        n170 = Equal?(x=w442, y="\u0010\u0000\u0002\u0000\u0002\u0016") -> (x = y?=w439:bool)
        n171 = Equal?(x=w442, y="å") -> (x = y?=w444:bool)
        n172 = Or(x=w440, y=w439) -> (x .or. y?=w438:bool)
        n173 = Or(x=w444, y=w438) -> (x .or. y?=w443:bool)
      }
      frame #3 {
        n174 = case shown="真" w472 {
          tunnel: [w474 w488] -> w469
          tunnel: [w473 w477] -> w468
          tunnel: w471 -> [w474 w479]
          tunnel: w470 -> [w473 w478]
          tunnel: [_ w476] -> w467
          tunnel: w466 -> [_ w475]
          frame False {
          }
          frame True {
            n175 = VISA Write(VISA resource name=w479, write buffer="\u0010\u0002\u0000\\^\u0016" ("写入缓冲区"), error in (no error)=w478) -> (VISA resource name out=w484:refnum<visa-resource-name>, error out=w481:errorcluster)  [unwired: 1 out]
            n176 = flat-sequence {
              tunnel: w484 -> [w491]
              tunnel: [w491] -> w483
              tunnel: [w490] -> w482
              tunnel: w481 -> [w490]
              tunnel: w475 -> [w489]
              frame #0 {
                n177 = local read "读写时间"() -> (w492:u32)
                n178 = Divide(x=w492, y=w489) -> (x/y=w493:dbl)
                n179 = Wait (ms)(milliseconds to wait=w493) -> ()  [unwired: 1 out]
              }
            }
            n180 = property class="Instr"(reference=w483, error in=w482) -> (reference out=w485:refnum<visa-resource-name>, error out=w487:errorcluster, "Serial Settings:Number of Bytes at Serial Port"=w486:u32)
            n181 = VISA Read(VISA resource name=w485, byte count=w486, error in (no error)=w487) -> (VISA resource name out=w488:refnum<visa-resource-name>, read buffer=w476:string, error out=w477:errorcluster)  [unwired: 1 out]
          }
        }
      }
      frame #4 {
        n182 = String Subset(string=w499, offset (0)=25 ("偏移量(0)"), length (rest)=4 ("长度（剩余）")) -> (substring=w502:string)
        n183 = String To Byte Array(string=w502) -> (unsigned byte array=w501:u8[])
        n184 = case shown="\"枚举RVW\"" w500 {
          tunnel: w501 -> [w505 w586 w667 _ _ _ _ _ _ _ _]
          tunnel: w499 -> [_ _ _ w749 _ _ _ _ _ _ _]
          frame "枚举RI" {
            n185 = stacked-sequence {
              seq-local: [w510 _ _ _] -> [_ w535 _ _]
              seq-local: [w508 _ _ _] -> [_ _ w552 _]
              seq-local: [w506 _ _ _] -> [_ _ _ w569]
              tunnel: w505 -> [w517 _ _ _]
              frame #0 {
                n186 = Index Array(array=w517, index=1 ("索引")) -> (element=w511:u8)
                n187 = Index Array(array=w517, index=2 ("索引")) -> (element=w509:u8)
                n188 = Index Array(array=w517, index=3 ("索引")) -> (element=w507:u8)
                n189 = Index Array(array=w517, index=0 ("索引")) -> (element=w512:u8)
                n190 = Number To Boolean Array(number=w511) -> (Boolean array=w510:bool[])
                n191 = Number To Boolean Array(number=w509) -> (Boolean array=w508:bool[])
                n192 = Number To Boolean Array(number=w507) -> (Boolean array=w506:bool[])
                n193 = Number To Boolean Array(number=w512) -> (Boolean array=w524:bool[])
                n194 = Index Array(array=w524, index=5 ("索引")) -> (element=→"I0.5":bool)
                n195 = Index Array(array=w524, index=6 ("索引")) -> (element=→"I0.6":bool)
                n196 = Index Array(array=w524, index=7 ("索引")) -> (element=→"I0.7":bool)
                n197 = Index Array(array=w524, index=2 ("索引")) -> (element=→"I0.2":bool)
                n198 = Index Array(array=w524, index=3 ("索引")) -> (element=→"I0.3":bool)
                n199 = Index Array(array=w524, index=4 ("索引")) -> (element=→"I0.4":bool)
                n200 = Index Array(array=w524, index=0 ("索引")) -> (element=→"I0.0":bool)
                n201 = Index Array(array=w524, index=1 ("索引")) -> (element=→"I0.1":bool)
              }
              frame #1 {
                n202 = Index Array(array=w535, index=1 ("索引")) -> (element=→"I1.1":bool)
                n203 = Index Array(array=w535, index=2 ("索引")) -> (element=→"I1.2":bool)
                n204 = Index Array(array=w535, index=7 ("索引")) -> (element=→"I1.7":bool)
                n205 = Index Array(array=w535, index=4 ("索引")) -> (element=→"I1.4":bool)
                n206 = Index Array(array=w535, index=6 ("索引")) -> (element=→"I1.6":bool)
                n207 = Index Array(array=w535, index=3 ("索引")) -> (element=→"I1.3":bool)
                n208 = Index Array(array=w535, index=0 ("索引")) -> (element=→"I1.0":bool)
                n209 = Index Array(array=w535, index=5 ("索引")) -> (element=→"I1.5":bool)
              }
              frame #2 {
                n210 = Index Array(array=w552, index=5 ("索引")) -> (element=→"I2.5":bool)
                n211 = Index Array(array=w552, index=6 ("索引")) -> (element=→"I2.6":bool)
                n212 = Index Array(array=w552, index=7 ("索引")) -> (element=→"I2.7":bool)
                n213 = Index Array(array=w552, index=2 ("索引")) -> (element=→"I2.2":bool)
                n214 = Index Array(array=w552, index=3 ("索引")) -> (element=→"I2.3":bool)
                n215 = Index Array(array=w552, index=4 ("索引")) -> (element=→"I2.4":bool)
                n216 = Index Array(array=w552, index=0 ("索引")) -> (element=→"I2.0":bool)
                n217 = Index Array(array=w552, index=1 ("索引")) -> (element=→"I2.1":bool)
              }
              frame #3 {
                n218 = Index Array(array=w569, index=1 ("索引")) -> (element=→"I3.1":bool)
                n219 = Index Array(array=w569, index=5 ("索引")) -> (element=→"I3.5":bool)
                n220 = Index Array(array=w569, index=6 ("索引")) -> (element=→"I3.6":bool)
                n221 = Index Array(array=w569, index=7 ("索引")) -> (element=→"I3.7":bool)
                n222 = Index Array(array=w569, index=2 ("索引")) -> (element=→"I3.2":bool)
                n223 = Index Array(array=w569, index=3 ("索引")) -> (element=→"I3.3":bool)
                n224 = Index Array(array=w569, index=4 ("索引")) -> (element=→"I3.4":bool)
                n225 = Index Array(array=w569, index=0 ("索引")) -> (element=→"I3.0":bool)
              }
            }
          }
          frame "枚举RQ" {
            n226 = stacked-sequence {
              seq-local: [w591 _ _ _] -> [_ w616 _ _]
              seq-local: [w589 _ _ _] -> [_ _ w633 _]
              seq-local: [w587 _ _ _] -> [_ _ _ w650]
              tunnel: w586 -> [w598 _ _ _]
              frame #0 {
                n227 = Index Array(array=w598, index=1 ("索引")) -> (element=w592:u8)
                n228 = Index Array(array=w598, index=2 ("索引")) -> (element=w590:u8)
                n229 = Index Array(array=w598, index=3 ("索引")) -> (element=w588:u8)
                n230 = Index Array(array=w598, index=0 ("索引")) -> (element=w593:u8)
                n231 = Number To Boolean Array(number=w592) -> (Boolean array=w591:bool[])
                n232 = Number To Boolean Array(number=w590) -> (Boolean array=w589:bool[])
                n233 = Number To Boolean Array(number=w588) -> (Boolean array=w587:bool[])
                n234 = Number To Boolean Array(number=w593) -> (Boolean array=w605:bool[])
                n235 = Index Array(array=w605, index=5 ("索引")) -> (element=→"Q0.5":bool)
                n236 = Index Array(array=w605, index=6 ("索引")) -> (element=→"Q0.6":bool)
                n237 = Index Array(array=w605, index=7 ("索引")) -> (element=→"Q0.7":bool)
                n238 = Index Array(array=w605, index=2 ("索引")) -> (element=→"Q0.2":bool)
                n239 = Index Array(array=w605, index=3 ("索引")) -> (element=→"Q0.3":bool)
                n240 = Index Array(array=w605, index=4 ("索引")) -> (element=→"Q0.4":bool)
                n241 = Index Array(array=w605, index=0 ("索引")) -> (element=→"Q0.0":bool)
                n242 = Index Array(array=w605, index=1 ("索引")) -> (element=→"Q0.1":bool)
              }
              frame #1 {
                n243 = Index Array(array=w616, index=1 ("索引")) -> (element=→"Q1.1":bool)
                n244 = Index Array(array=w616, index=2 ("索引")) -> (element=→"Q1.2":bool)
                n245 = Index Array(array=w616, index=7 ("索引")) -> (element=→"Q1.7":bool)
                n246 = Index Array(array=w616, index=4 ("索引")) -> (element=→"Q1.4":bool)
                n247 = Index Array(array=w616, index=6 ("索引")) -> (element=→"Q1.6":bool)
                n248 = Index Array(array=w616, index=3 ("索引")) -> (element=→"Q1.3":bool)
                n249 = Index Array(array=w616, index=0 ("索引")) -> (element=→"Q1.0":bool)
                n250 = Index Array(array=w616, index=5 ("索引")) -> (element=→"Q1.5":bool)
              }
              frame #2 {
                n251 = Index Array(array=w633, index=5 ("索引")) -> (element=→"Q2.5":bool)
                n252 = Index Array(array=w633, index=6 ("索引")) -> (element=→"Q2.6":bool)
                n253 = Index Array(array=w633, index=7 ("索引")) -> (element=→"Q2.7":bool)
                n254 = Index Array(array=w633, index=2 ("索引")) -> (element=→"Q2.2":bool)
                n255 = Index Array(array=w633, index=3 ("索引")) -> (element=→"Q2.3":bool)
                n256 = Index Array(array=w633, index=4 ("索引")) -> (element=→"Q2.4":bool)
                n257 = Index Array(array=w633, index=0 ("索引")) -> (element=→"Q2.0":bool)
                n258 = Index Array(array=w633, index=1 ("索引")) -> (element=→"Q2.1":bool)
              }
              frame #3 {
                n259 = Index Array(array=w650, index=1 ("索引")) -> (element=→"Q3.1":bool)
                n260 = Index Array(array=w650, index=5 ("索引")) -> (element=→"Q3.5":bool)
                n261 = Index Array(array=w650, index=6 ("索引")) -> (element=→"Q3.6":bool)
                n262 = Index Array(array=w650, index=7 ("索引")) -> (element=→"Q3.7":bool)
                n263 = Index Array(array=w650, index=2 ("索引")) -> (element=→"Q3.2":bool)
                n264 = Index Array(array=w650, index=3 ("索引")) -> (element=→"Q3.3":bool)
                n265 = Index Array(array=w650, index=4 ("索引")) -> (element=→"Q3.4":bool)
                n266 = Index Array(array=w650, index=0 ("索引")) -> (element=→"Q3.0":bool)
              }
            }
          }
          frame "枚举RM" {
            n267 = stacked-sequence {
              seq-local: [w673 _ _ _] -> [_ w697 _ _]
              seq-local: [w671 _ _ _] -> [_ _ w714 _]
              seq-local: [w669 _ _ _] -> [_ _ _ w731]
              tunnel: w667 -> [w668 _ _ _]
              frame #0 {
                n268 = Index Array(array=w668, index=1 ("索引")) -> (element=w674:u8)
                n269 = Index Array(array=w668, index=2 ("索引")) -> (element=w672:u8)
                n270 = Index Array(array=w668, index=3 ("索引")) -> (element=w670:u8)
                n271 = Index Array(array=w668, index=0 ("索引")) -> (element=w675:u8)
                n272 = Number To Boolean Array(number=w674) -> (Boolean array=w673:bool[])
                n273 = Number To Boolean Array(number=w672) -> (Boolean array=w671:bool[])
                n274 = Number To Boolean Array(number=w670) -> (Boolean array=w669:bool[])
                n275 = Number To Boolean Array(number=w675) -> (Boolean array=w686:bool[])
                n276 = Index Array(array=w686, index=6 ("索引")) -> (element=→"M0.6":bool)
                n277 = Index Array(array=w686, index=7 ("索引")) -> (element=→"M0.7":bool)
                n278 = Index Array(array=w686, index=2 ("索引")) -> (element=→"M0.2":bool)
                n279 = Index Array(array=w686, index=3 ("索引")) -> (element=→"M0.3":bool)
                n280 = Index Array(array=w686, index=4 ("索引")) -> (element=→"M0.4":bool)
                n281 = Index Array(array=w686, index=0 ("索引")) -> (element=→"M0.0":bool)
                n282 = Index Array(array=w686, index=1 ("索引")) -> (element=→"M0.1":bool)
                n283 = Index Array(array=w686, index=5 ("索引")) -> (element=→"M0.5":bool)
              }
              frame #1 {
                n284 = Index Array(array=w697, index=1 ("索引")) -> (element=→"M1.1":bool)
                n285 = Index Array(array=w697, index=2 ("索引")) -> (element=→"M1.2":bool)
                n286 = Index Array(array=w697, index=7 ("索引")) -> (element=→"M1.7":bool)
                n287 = Index Array(array=w697, index=4 ("索引")) -> (element=→"M1.4":bool)
                n288 = Index Array(array=w697, index=6 ("索引")) -> (element=→"M1.6":bool)
                n289 = Index Array(array=w697, index=3 ("索引")) -> (element=→"M1.3":bool)
                n290 = Index Array(array=w697, index=0 ("索引")) -> (element=→"M1.0":bool)
                n291 = Index Array(array=w697, index=5 ("索引")) -> (element=→"M1.5":bool)
              }
              frame #2 {
                n292 = Index Array(array=w714, index=5 ("索引")) -> (element=→"M2.5":bool)
                n293 = Index Array(array=w714, index=6 ("索引")) -> (element=→"M2.6":bool)
                n294 = Index Array(array=w714, index=7 ("索引")) -> (element=→"M2.7":bool)
                n295 = Index Array(array=w714, index=2 ("索引")) -> (element=→"M2.2":bool)
                n296 = Index Array(array=w714, index=3 ("索引")) -> (element=→"M2.3":bool)
                n297 = Index Array(array=w714, index=4 ("索引")) -> (element=→"M2.4":bool)
                n298 = Index Array(array=w714, index=0 ("索引")) -> (element=→"M2.0":bool)
                n299 = Index Array(array=w714, index=1 ("索引")) -> (element=→"M2.1":bool)
              }
              frame #3 {
                n300 = Index Array(array=w731, index=1 ("索引")) -> (element=→"Q3.1":bool)
                n301 = Index Array(array=w731, index=5 ("索引")) -> (element=→"Q3.5":bool)
                n302 = Index Array(array=w731, index=6 ("索引")) -> (element=→"Q3.6":bool)
                n303 = Index Array(array=w731, index=7 ("索引")) -> (element=→"Q3.7":bool)
                n304 = Index Array(array=w731, index=2 ("索引")) -> (element=→"Q3.2":bool)
                n305 = Index Array(array=w731, index=3 ("索引")) -> (element=→"Q3.3":bool)
                n306 = Index Array(array=w731, index=4 ("索引")) -> (element=→"Q3.4":bool)
                n307 = Index Array(array=w731, index=0 ("索引")) -> (element=→"Q3.0":bool)
              }
            }
          }
          frame "枚举RVW" {
            n308 = String Subset(string=w749, offset (0)=25 ("偏移量(0)"), length (rest)=40 ("长度（剩余）")) -> (substring=w748:string)
            n309 = stacked-sequence {
              tunnel: w748 -> [w752 w807]
              frame #0 {
                n310 = String Subset(string=w752, offset (0)=6 ("偏移量(0)"), length (rest)=8 ("长度（剩余）")) -> (substring=w784:string)
                n311 = String Subset(string=w752, offset (0)=0 ("偏移量(0)"), length (rest)=2 ("长度（剩余）")) -> (substring=w793:string)
                n312 = String Subset(string=w752, offset (0)=2 ("偏移量(0)"), length (rest)=4 ("长度（剩余）")) -> (substring=w792:string)
                n313 = String Subset(string=w752, offset (0)=4 ("偏移量(0)"), length (rest)=6 ("长度（剩余）")) -> (substring=w785:string)
                n314 = String Subset(string=w752, offset (0)=8 ("偏移量(0)"), length (rest)=10 ("长度（剩余）")) -> (substring=w777:string)
                n315 = String Subset(string=w752, offset (0)=16 ("偏移量(0)"), length (rest)=18 ("长度（剩余）")) -> (substring=w755:string)
                n316 = String Subset(string=w752, offset (0)=10 ("偏移量(0)"), length (rest)=12 ("长度（剩余）")) -> (substring=w776:string)
                n317 = String Subset(string=w752, offset (0)=12 ("偏移量(0)"), length (rest)=14 ("长度（剩余）")) -> (substring=w769:string)
                n318 = String Subset(string=w752, offset (0)=14 ("偏移量(0)"), length (rest)=16 ("长度（剩余）")) -> (substring=w768:string)
                n319 = Type Cast(type=u16 0, x=w784) -> (*(type *) &x=→"RVW6":u16)
                n320 = Type Cast(type=u16 0, x=w793) -> (*(type *) &x=→"RVW0":u16)
                n321 = Type Cast(type=u16 0, x=w792) -> (*(type *) &x=→"RVW2":u16)
                n322 = Type Cast(type=u16 0, x=w785) -> (*(type *) &x=→"RVW4":u16)
                n323 = Type Cast(type=u16 0, x=w777) -> (*(type *) &x=→"RVW8":u16)
                n324 = Type Cast(type=u16 0, x=w755) -> (*(type *) &x=→"RVW16":u16)
                n325 = Type Cast(type=u16 0, x=w776) -> (*(type *) &x=→"RVW10":u16)
                n326 = Type Cast(type=u16 0, x=w769) -> (*(type *) &x=→"RVW12":u16)
                n327 = Type Cast(type=u16 0, x=w768) -> (*(type *) &x=→"RVW14":u16)
              }
              frame #1 {
                n328 = String Subset(string=w807, offset (0)=18 ("偏移量(0)"), length (rest)=20 ("长度（剩余）")) -> (substring=w840:string)
                n329 = String Subset(string=w807, offset (0)=20 ("偏移量(0)"), length (rest)=22 ("长度（剩余）")) -> (substring=w839:string)
                n330 = String Subset(string=w807, offset (0)=22 ("偏移量(0)"), length (rest)=24 ("长度（剩余）")) -> (substring=w832:string)
                n331 = String Subset(string=w807, offset (0)=24 ("偏移量(0)"), length (rest)=26 ("长度（剩余）")) -> (substring=w831:string)
                n332 = String Subset(string=w807, offset (0)=26 ("偏移量(0)"), length (rest)=28 ("长度（剩余）")) -> (substring=w824:string)
                n333 = String Subset(string=w807, offset (0)=28 ("偏移量(0)"), length (rest)=30 ("长度（剩余）")) -> (substring=w823:string)
                n334 = String Subset(string=w807, offset (0)=30 ("偏移量(0)"), length (rest)=32 ("长度（剩余）")) -> (substring=w816:string)
                n335 = String Subset(string=w807, offset (0)=32 ("偏移量(0)"), length (rest)=34 ("长度（剩余）")) -> (substring=w815:string)
                n336 = String Subset(string=w807, offset (0)=34 ("偏移量(0)"), length (rest)=36 ("长度（剩余）")) -> (substring=w808:string)
                n337 = Type Cast(type=u16 0, x=w840) -> (*(type *) &x=→"RVW18":u16)
                n338 = Type Cast(type=u16 0, x=w839) -> (*(type *) &x=→"RVW20":u16)
                n339 = Type Cast(type=u16 0, x=w832) -> (*(type *) &x=→"RVW22":u16)
                n340 = Type Cast(type=u16 0, x=w831) -> (*(type *) &x=→"RVW24":u16)
                n341 = Type Cast(type=u16 0, x=w824) -> (*(type *) &x=→"RVW26":u16)
                n342 = Type Cast(type=u16 0, x=w823) -> (*(type *) &x=→"RVW28":u16)
                n343 = Type Cast(type=u16 0, x=w816) -> (*(type *) &x=→"RVW30":u16)
                n344 = Type Cast(type=u16 0, x=w815) -> (*(type *) &x=→"RVW32":u16)
                n345 = Type Cast(type=u16 0, x=w808) -> (*(type *) &x=→"RVW34":u16)
              }
            }
          }
          frame "WID0" {
          }
          frame "WQD0" {
          }
          frame "WMD0" {
          }
          frame "WV" {
          }
          frame "STOP" {
          }
          frame "RUN" {
          }
          frame "捂手" {
          }
        }
      }
    }
  }
  n346 = VISA Flush I/O Buffer(VISA resource name=w7, error in (no error)=w6) -> (VISA resource name out=w5:refnum<visa-resource-name>, error out=w4:errorcluster)  [unwired: 1 in]
  n347 = VISA Close(VISA resource name=w5, error in (no error)=w4) -> ()  [unwired: 1 out]
